vi "ResetAngleWithOffsetFunction.vi"(10 "Offset":dbl, 11 "AngleInput":dbl) -> (3 "AngleOutput":dbl)   [LabVIEW 2017]
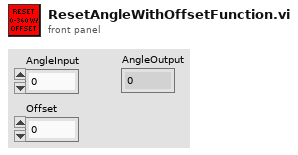
[diagram p1: front panel]
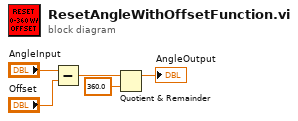
[diagram p0: block diagram]
diagram:
  n1 = Subtract(x="AngleInput", y="Offset") -> (x-y=w2:dbl)
  n2 = Quotient & Remainder(x=w2, y=360.0) -> (x-y*floor(x/y)=→"AngleOutput":dbl)  [unwired: 1 out]
